vi "while loop.vi"() -> ()   [LabVIEW 2014]
panel:
  out "output":dbl format="%#_13g"
  in  "input":dbl format="%#_13g"
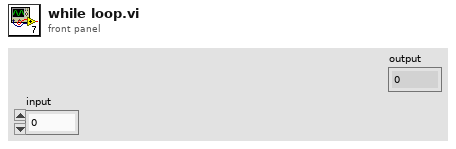
[diagram p1: front panel]
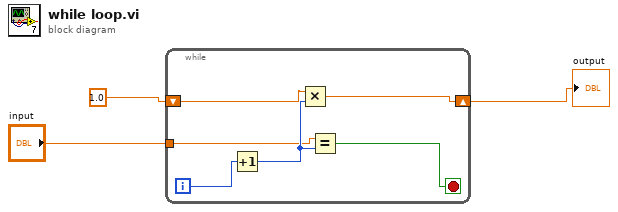
[diagram p0: block diagram]
diagram:
  n1 = while {
    tunnel: "input" -> [w6]
    shift-right: [w4] -> w2
    shift-left: 1.0 -> [w5]
    i -> [w8]
    stop <- w7 stop-if-true
    n2 = Increment(x=w8) -> (x+1=w9:i32)
    n3 = Multiply(x=w5, y=w9) -> (x*y=w4:dbl)
    n4 = Equal?(x=w6, y=w9) -> (x = y?=w7:bool)
  }
  "output" <- w2
